vi "Jesper.vi"(9 "REPL":string, 10 "Send":string) -> ()   [LabVIEW 2020]
panel:
  in  "start pybricks":bool
  out "Cover":bool
  in  "Script":string
  in  "Buffer":string
  in  "Disconnect":bool
  in  "EV3":T1={"rPi IP Address"="192.168.1.19", "Username"="robot", "password"="maker"}
  in  "Help":bool
  in  "Connect":bool
  in  "Stop Button":bool
  out "Running Script":bool
  in  "Abort":bool
  in  "xPort":string
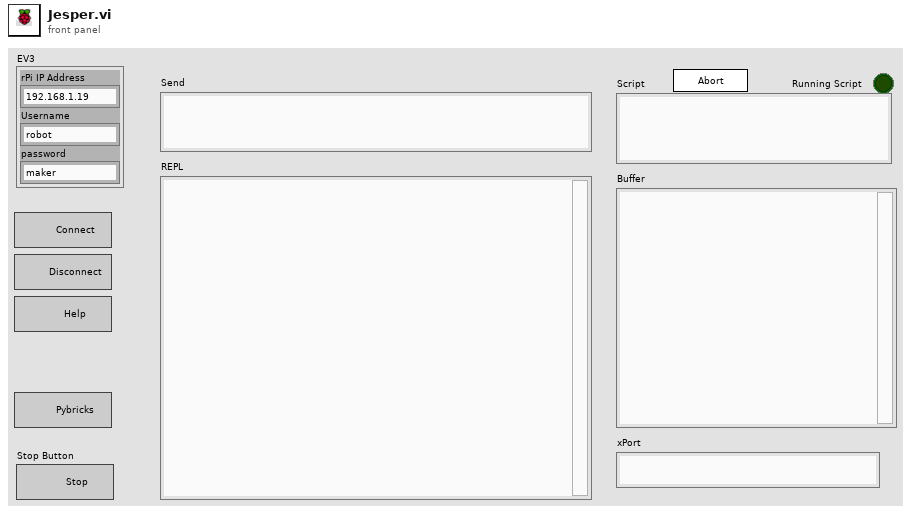
[diagram p1: front panel]
types:
  T1 = cluster{"rPi IP Address":string, "Username":string, "password":string}
  T2 = enum32{"Invalid", "Standard", "Closed", "Hidden", "Minimized", "Maximized"}
  T3 = typedef "eventvkey.ctl" = enum16{"ASCII", "Enter", "Return", "Shift", "Ctrl", "Alt", "Cmd", "Opt", "Caps", "NumLock", "Clear", "Break", "Up", "Down", "Left", "Right", "Insert", "Delete", "Home", "End", "PageUp", "PageDown", "Escape", "Help", "Pause", "ScrollLock", "F1", "F2", "F3", "F4", "F5", "F6", "F7", "F8", "F9", "F10", "F11", "F12", "F13", "F14", "F15", "F16", "F17", "F18", "F19", "F20", "F21", "F22", "F23", "F24", "Play", "VolumeUp", "VolumeDown", "Mute", "Two Byte Char"}
  T4 = cluster{"Shift":bool, "Ctrl":bool, "Alt":bool, "Cmd":bool, "Opt":bool}
  T5 = cluster{"Char":i16, "VKey":T3, "PlatMods":cluster{"Shift":bool, "Ctrl":bool, "Alt":bool, "Cmd":bool, "Opt":bool}}
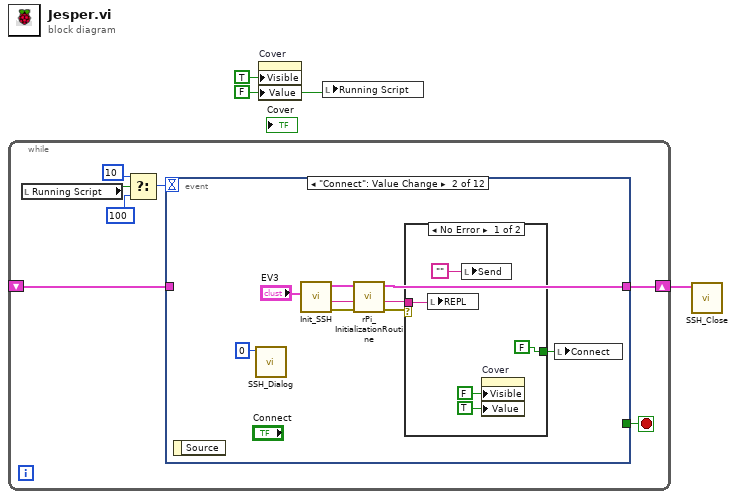
[diagram p0: block diagram]
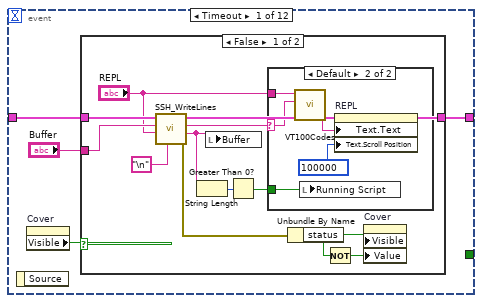
[diagram p2: hidden frame]
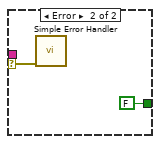
[diagram p5: hidden frame]
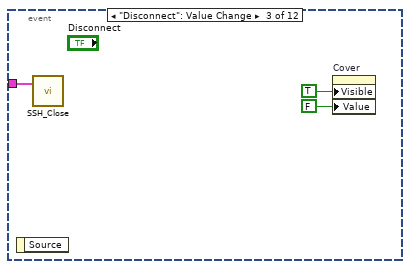
[diagram p6: hidden frame]
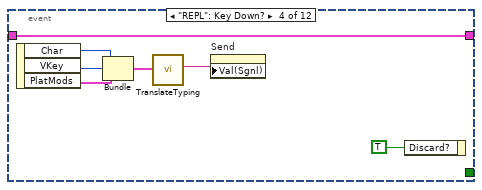
[diagram p7: hidden frame]
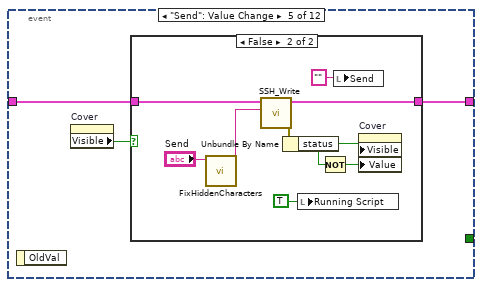
[diagram p8: hidden frame]
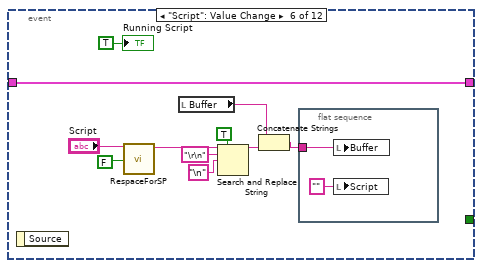
[diagram p10: hidden frame]
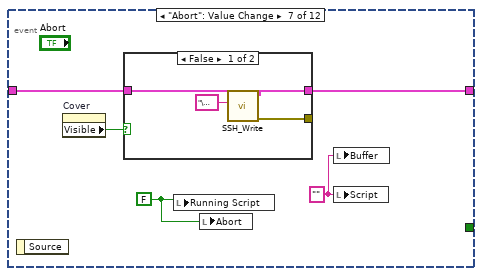
[diagram p11: hidden frame]
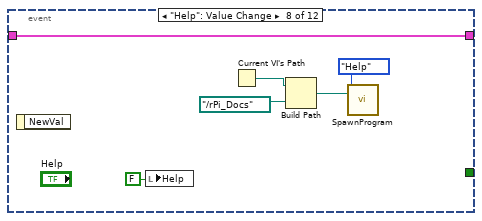
[diagram p13: hidden frame]
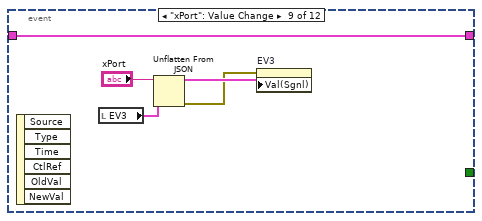
[diagram p14: hidden frame]
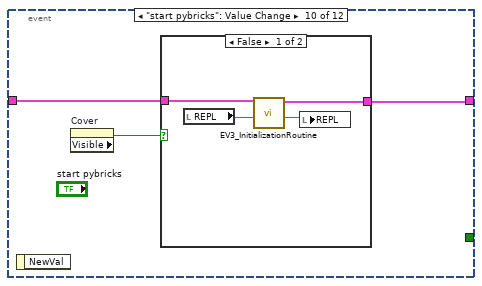
[diagram p15: hidden frame]
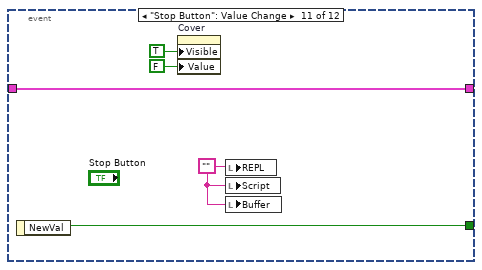
[diagram p17: hidden frame]
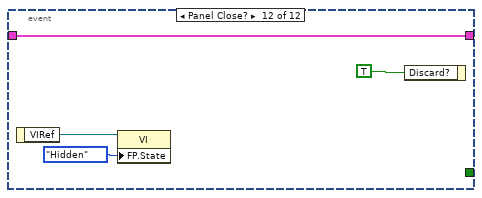
[diagram p18: hidden frame]
diagram:
  w1 = FALSE ("Cover")
  n1 = while {
    shift-right: [w9] -> w2
    shift-left: _ -> [w8]
    stop <- w10 stop-if-true
    n2 = local read "Running Script"() -> (w4:bool)
    n3 = Select(t=10, s=w4, f=100) -> (s? t:f=w5:i32)
    n4 = event shown="[1] \"Connect\": Value Change" {
      selector: _ -> [_ _ _ _ _ _ _ _ _ _ _ _]
      dyn-events: _ -> [_ _ _ _ _ _ _ _ _ _ _ _]
      timeout: w5 -> [_ _ _ _ _ _ _ _ _ _ _ _]
      tunnel: [_ _ _ _ _ _ _ _ _ _ w117 _] -> w10
      tunnel: [w14 w35 _ w57 w60 w82 w87 w100 w105 w106 w118 w122] -> w9
      tunnel: w8 -> [w12 _ w51 w57 w61 w82 w88 w100 w105 w107 w118 w122]
      event Timeout {
        n5 = event-data() -> ()  [unwired: 1 in, 1 out]
        n6 = property on="Cover" class="Bool (strict)"() -> ("Visible"=w13:bool)  [unwired: 2 in, 2 out]
        n7 = case shown="False" w13 {
          tunnel: [w24 w32] -> w14
          tunnel: w12 -> [w26 w32]
          tunnel: "Buffer" -> [w25 _]
          frame False {
            n8 = call "SSH_WriteLines.vi"("search char"="\n" ("search string"), "REPL"="REPL", "Buffer"=w25, "Python in"=w26) -> ("error out"=w21:errorcluster, "Rest"=w19:string, "Reply"=w23:string, "Python out"=w24:cluster{"Python":refnum<k35>, "py file":path})  [unwired: 4 in]
            n9 = String Length(string=w19) -> (length=w20:i32)
            n10 = local write "Buffer"(w19) -> ()
            n11 = Greater Than 0?(x=w20) -> (x > 0?=w18:bool)
            n12 = case shown="Default" w23 {
              selector: w23 -> [_ w28]
              tunnel: "REPL" -> [_ w29]
              tunnel: w18 -> [_ w27]
              frame "" {
              }
              frame Default {
                n13 = call "VT100Codes.vi"("read buffer"=w28, "Console In"=w29) -> ("Console Out"=w30:string)  [unwired: 9 in]
                n14 = local write "Running Script"(w27) -> ()
                n15 = property on="REPL" class="Str"("Text.Text"=w30, "Text.Scroll Position"=u32 100000 ("Text.Selection:Start")) -> ()  [unwired: 2 in, 2 out]
              }
            }
            n16 = Unbundle By Name(w21) -> ("status"=w16:bool)
            n17 = Not(x=w16) -> (.not. x?=w15:bool)
            n18 = property on="Cover" class="Bool (strict)"("Visible"=w16, "Value"=w15) -> ()  [unwired: 2 in, 2 out]
          }
          frame True {
          }
        }
      }
      event "Connect": Value Change {
        n19 = event-data() -> ()  [unwired: 1 in, 1 out]
        n20 = call "SSH_Dialog.vi"("Slide"=u8 0) -> ()  [unwired: 11 in]
        n21 = call "Init_SSH.vi"("EV3"="EV3") -> ("error out"=w34:errorcluster, "Console out"=w33:string, "Python out"=w36:cluster{"Python":refnum<k35>, "py file":path})  [unwired: 8 in]
        n22 = call "rPi_InitializationRoutine.vi"("error in (no error)"=w34, "Console In"=w33, "Python in"=w36) -> ("error out"=w38:errorcluster, "Console Out"=w37:string, "Python out"=w35:cluster{"Python":refnum<k35>, "py file":path})  [unwired: 6 in]
        n23 = case shown="No Error" w38 {
          selector: w38 -> [_ w48]
          tunnel: w37 -> [w43 _]
          tunnel: [FALSE ("Cover") FALSE ("Cover")] -> w39
          frame No Error {
            n24 = local write "REPL"(w43) -> ()
            n25 = local write "Send"("") -> ()
            n26 = property on="Cover" class="Bool (strict)"("Visible"=FALSE, "Value"=TRUE ("Cover")) -> ()  [unwired: 2 in, 2 out]
          }
          frame Error {
            n27 = call <vilib>:"Simple Error Handler.vi"("error in (no error)"=w48) -> ()  [unwired: 4 in, 5 out]
          }
        }
        n28 = local write "Connect"(w39) -> ()
      }
      event "Disconnect": Value Change {
        n29 = event-data() -> ()  [unwired: 1 in, 1 out]
        n30 = call "SSH_Close.vi"("Python in"=w51) -> ()  [unwired: 11 in]
        n31 = property on="Cover" class="Bool (strict)"("Visible"=TRUE, "Value"=FALSE ("Cover")) -> ()  [unwired: 2 in, 2 out]
      }
      event "REPL": Key Down? {
        n32 = event-data() -> ("Char"=w55:i16, "VKey"=w54:T3, "PlatMods"=w53:T4)  [unwired: 1 in]
        n33 = Bundle("Char"=w55, "VKey"=w54, "PlatMods"=w53) -> (w56:T5)  [unwired: 1 in]
        n34 = call "TranslateTyping.vi"("Cluster"=w56) -> ("key"=w52:string)  [unwired: 10 in]
        n35 = property on="Send" class="Str"("Val(Sgnl)"=w52) -> ()  [unwired: 2 in, 2 out]
        n36 = event-data("Discard?"=TRUE) -> ()  [unwired: 1 in, 1 out]
      }
      event "Send": Value Change {
        n37 = event-data() -> ()  [unwired: 1 in, 1 out]
        n38 = property on="Cover" class="Bool (strict)"() -> ("Visible"=w59:bool)  [unwired: 2 in, 2 out]
        n39 = case shown="False" w59 {
          tunnel: w61 -> [w62 w70]
          tunnel: [w62 w69] -> w60
          frame True {
          }
          frame False {
            n40 = call "FixHiddenCharacters.vi"("String in"="Send") -> ("String out"=w67:string)  [unwired: 10 in]
            n41 = call "SSH_Write.vi"("Text to write"=w67, "Python in"=w70) -> ("error out"=w63:errorcluster, "Python out"=w69:cluster{"Python":refnum<k35>, "py file":path})  [unwired: 8 in]
            n42 = Unbundle By Name(w63) -> ("status"=w65:bool)
            n43 = local write "Running Script"(TRUE ("Running Script")) -> ()
            n44 = Not(x=w65) -> (.not. x?=w64:bool)
            n45 = local write "Send"("" ("Write text")) -> ()
            n46 = property on="Cover" class="Bool (strict)"("Visible"=w65, "Value"=w64) -> ()  [unwired: 2 in, 2 out]
          }
        }
      }
      event "Script": Value Change {
        n47 = event-data() -> ()  [unwired: 1 in, 1 out]
        n48 = call "RespaceForSP.vi"("Keep spaces?"=FALSE, "Code"="Script") -> ("Cleaned for SPIKE"=w77:string)  [unwired: 9 in]
        n49 = local read "Buffer"() -> (w74:string)
        n50 = Search and Replace String(replace all?=TRUE ("replace all? (F)"), input string=w77, search string="\r\n", replace string="\n" ("search string")) -> (result string=w73:string)  [unwired: 4 in, 3 out]
        n51 = Concatenate Strings(w74, w73) -> (w72:string)
        n52 = flat-sequence {
          tunnel: w72 -> [w84]
          frame #0 {
            n53 = local write "Buffer"(w84) -> ()
            n54 = local write "Script"("" ("Script")) -> ()
          }
        }
        "Running Script" <- TRUE ("Running Script")
      }
      event "Abort": Value Change {
        w89 = "" ("Script")
        w86 = FALSE ("Running Script")
        n55 = event-data() -> ()  [unwired: 1 in, 1 out]
        n56 = property on="Cover" class="Bool (strict)"() -> ("Visible"=w85:bool)  [unwired: 2 in, 2 out]
        n57 = case shown="False" w85 {
          tunnel: w88 -> [w93 w94]
          tunnel: [w92 w94] -> w87
          tunnel: [w90 _] -> _
          frame False {
            n58 = call "SSH_Write.vi"("Text to write"="\u0003", "Python in"=w93) -> ("error out"=w90:errorcluster, "Python out"=w92:cluster{"Python":refnum<k35>, "py file":path})  [unwired: 8 in]
          }
          frame True {
          }
        }
        n59 = local write "Running Script"(w86) -> ()
        n60 = local write "Abort"(w86) -> ()
        n61 = local write "Buffer"(w89) -> ()
        n62 = local write "Script"(w89) -> ()
      }
      event "Help": Value Change {
        n63 = event-data() -> ()  [unwired: 1 in, 1 out]
        n64 = local write "Help"(FALSE ("Help")) -> ()
        n65 = Current VI's Path() -> (path=w98:path)
        n66 = Build Path(base path=w98, name or relative path=path "../rPi_Docs") -> (appended path=w95:path)
        n67 = call "SpawnProgram.vi"("Server"=w95, "Dialog"=enum16{"Help", "Files"}."Help") -> ()  [unwired: 10 in]
      }
      event "xPort": Value Change {
        n68 = event-data() -> ()  [unwired: 1 in, 6 out]
        n69 = local read "EV3"() -> (w101:T1)
        n70 = Unflatten From JSON(JSON string="xPort", type and defaults=w101) -> (value=w103:T1, error out=w102:errorcluster)  [unwired: 5 in]
        n71 = property on="EV3" class="Clust (strict)"(error in=w102, "Val(Sgnl)"=w103) -> ()  [unwired: 1 in, 2 out]
      }
      event "start pybricks": Value Change {
        n72 = event-data() -> ()  [unwired: 1 in, 1 out]
        n73 = property on="Cover" class="Bool (strict)"() -> ("Visible"=w108:bool)  [unwired: 2 in, 2 out]
        n74 = case shown="False" w108 {
          tunnel: w107 -> [w111 w113]
          tunnel: [w112 w113] -> w106
          frame False {
            n75 = local read "REPL"() -> (w110:string)
            n76 = call "EV3_InitializationRoutine.vi"("Console In"=w110, "Python in"=w111) -> ("Console Out"=w109:string, "Python out"=w112:cluster{"Python":refnum<k35>, "py file":path})  [unwired: 7 in, 1 out]
            n77 = local write "REPL"(w109) -> ()
          }
          frame True {
          }
        }
      }
      event "Stop Button": Value Change {
        w114 = ""
        n78 = event-data() -> ("NewVal"=w117:bool)  [unwired: 1 in]
        n79 = property on="Cover" class="Bool (strict)"("Visible"=TRUE, "Value"=FALSE ("Cover")) -> ()  [unwired: 2 in, 2 out]
        n80 = local write "REPL"(w114) -> ()
        n81 = local write "Script"(w114) -> ()
        n82 = local write "Buffer"(w114) -> ()
      }
      event Panel Close? {
        n83 = event-data() -> ("VIRef"=w120:refnum<vi>)  [unwired: 1 in]
        n84 = property class="VI"(reference=w120, "FP.State"=T2."Hidden" ("Front Panel Window:State")) -> ()  [unwired: 1 in, 2 out]
        n85 = event-data("Discard?"=TRUE) -> ()  [unwired: 1 in, 1 out]
      }
    }
  }
  n86 = property on="Cover" class="Bool (strict)"("Visible"=TRUE, "Value"=w1) -> ()  [unwired: 2 in, 2 out]
  n87 = local write "Running Script"(w1) -> ()
  n88 = call "SSH_Close.vi"("Python in"=w2) -> ()  [unwired: 11 in]
